vi "Cleanup.vi"(8 "error in (no error)":errorcluster, 11 "AppListPanel in":refnum<class "AppListPanel.lvclass">) -> (0 "error out":errorcluster)   [LabVIEW 2020, in "PicoG-App.lvlib" / "AppListPanel.lvclass"]
uses:
  AppListPanel.lvclass
  AppListPanel.lvclass/AppListPanel.ctl
  <vilib>/IlluminatedG/IG OOPanel/OOPanel/Panel/Panel.lvclass
  <vilib>/IlluminatedG/IG OOPanel/OOPanel/ArrayManager/ArrayManager.lvclass
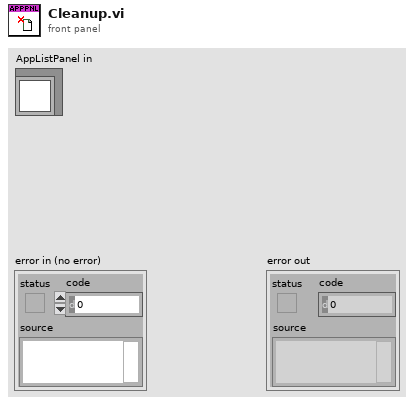
[diagram p1: front panel]
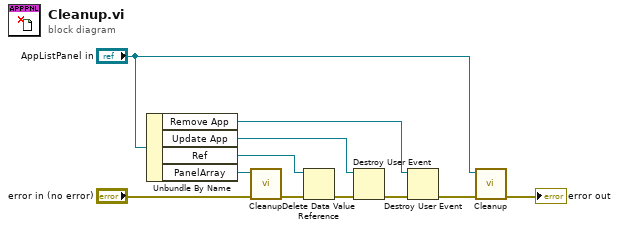
[diagram p0: block diagram]
diagram:
  n1 = Unbundle By Name("AppListPanel in") -> ("Remove App"=w3:refnum<user-event>, "Update App"=w4:refnum<user-event>, "Ref"=w7:refnum<data-value>, "PanelArray"=w8:refnum<class "ArrayManager.lvclass">)
  n2 = call <vilib>:"Cleanup.vi"("error in (no error)"="error in (no error)", "PanelArray in"=w8) -> ("error out"=w6:errorcluster)  [unwired: 9 in]
  n3 = Delete Data Value Reference(data value reference=w7, error in=w6) -> (error out=w5:errorcluster)  [unwired: 1 out]
  n4 = Destroy User Event(user event=w4, error in=w5) -> (error out=w2:errorcluster)
  n5 = Destroy User Event(user event=w3, error in=w2) -> (error out=w1:errorcluster)
  n6 = call-parent <vilib>:"Cleanup.vi"("error in (no error)"=w1, "Panel in"="AppListPanel in") -> ("error out"=→"error out":errorcluster)  [unwired: 9 in]
